vi "Update.vi"(8 "error in (no error)":errorcluster, 10 "Simulation Objects in":refnum<class "SimulationObject.lvclass">[](array[class]), 11 "Updatable in":refnum<class "Updatable.lvclass">) -> (0 "error out":errorcluster, 2 "Simulation Objects out":refnum<class "SimulationObject.lvclass">[](array[class]), 3 "Updatable out":refnum<class "Updatable.lvclass">)   [LabVIEW 2022 SP3, in "Updatable.lvclass"]
uses:
  Updatable.lvclass
  Objects/SimulationObject/SimulationObject.lvclass
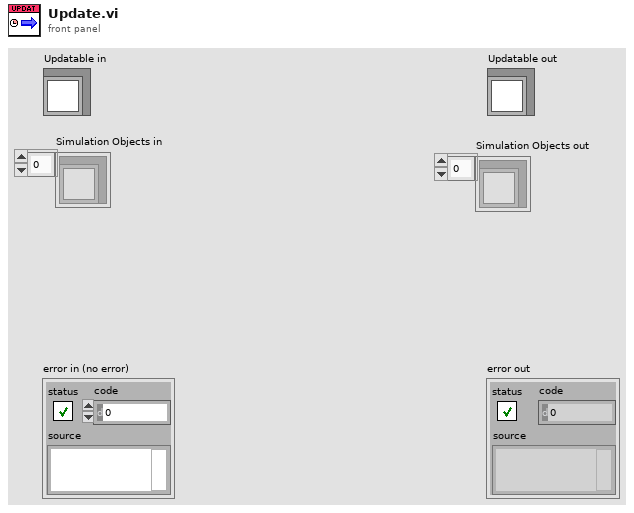
[diagram p1: front panel]
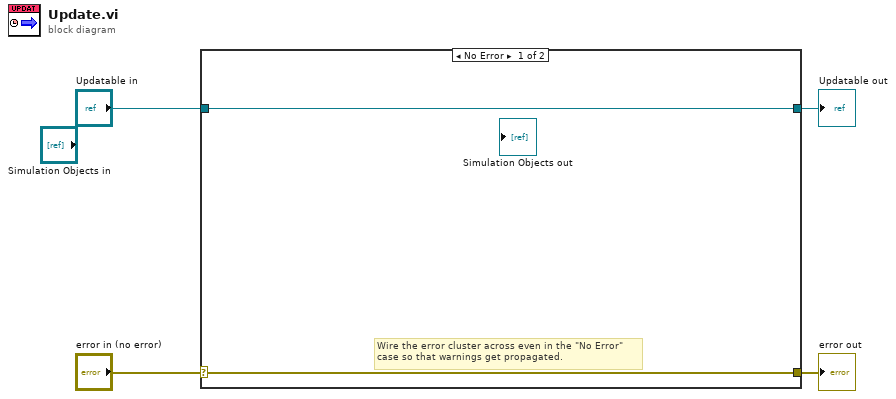
[diagram p0: block diagram]
diagram:
  n1 = case shown="No Error" "error in (no error)" {
    selector: "error in (no error)" -> [w5 w8]
    tunnel: [w5 w8] -> w3
    tunnel: [w6 w7] -> w1
    tunnel: "Updatable in" -> [w6 w7]
    frame No Error {
      # "Wire the error cluster across even in the \"No Error\"\ncase so that warnings get propagated."
    }
    frame Error {
    }
  }
  "error out" <- w3
  "Updatable out" <- w1
